vi "download_device_list_extended.vi"(8 "configuration":u64, 9 "port":u16, 10 "host":string, 11 "path in":path=path "hl2ss_ulm.dll") -> (2 "error":bool, 3 "utf16_string":u8[](array[numeric]))   [LabVIEW 2023]
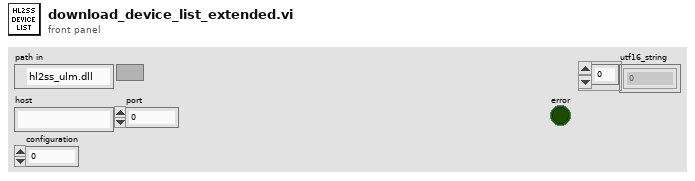
[diagram p1: front panel]
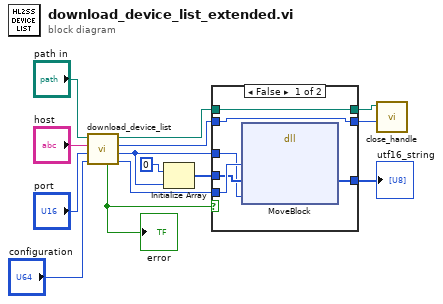
[diagram p0: block diagram]
diagram:
  n1 = call "download_device_list.vi"("configuration"="configuration", "port"="port", "host"="host", "path in"="path in") -> ("query"=w9:u64, "size"=w7:u64, "device_list_handle"=w6:u64, "path out"=w5:path, "error"=w10:bool)  [unwired: 3 in]
  "error" <- w10
  n2 = Initialize Array(u8 0 ("element"), w7) -> (w8:u8[])
  n3 = case shown="False" w10 {
    tunnel: w9 -> [w20 _]
    tunnel: w8 -> [w19 w21]
    tunnel: w7 -> [w18 _]
    tunnel: w6 -> [w16 w23]
    tunnel: w5 -> [w17 w22]
    tunnel: [w17 w22] -> w4
    tunnel: [w16 w23] -> w3
    tunnel: [w15 w21] -> w2
    frame False {
      n4 = dll-call lib="LabVIEW" fn="MoveBlock"("ps"=w20, "pd"=w19, "size"=w18) -> ("pd"=w15:u8[])  [unwired: 6 in, 2 out]
    }
    frame True {
    }
  }
  "utf16_string" <- w2
  n5 = call "close_handle.vi"("handle"=w3, "path in"=w4) -> ()  [unwired: 9 in, 1 out]
